vi "Intan_FilterSettings.vi"(0 "VISA resource name":refnum<visa-resource-name>="COM1", 1 "R_L source":u8(ring) items=["ON-chip", "OFF-chip"], 2 "Lower cutoff":u8(ring)=12 items=["10 Hz", "7.5 Hz", "5.0 Hz", "3.0 Hz", "2.5 Hz", "2.0 Hz", "1.5 Hz", "1.0 Hz", "0.75 Hz", "0.5 Hz", "0.3 Hz", "0.25 Hz", "0.10 Hz"], 3 "Upper cutoff":u8(ring)=10 items=["5.0 kHz", "3.0 kHz", "2.5 kHz", "2.0 kHz", "1.5 kHz", "1.0 kHz", "750 Hz", "500 Hz", "300 Hz", "250 Hz", "200 Hz", "150 Hz", "100 Hz"], 4 "error in":errorcluster) -> (5 "VISA resource name out":refnum<visa-resource-name>, 6 "Text response":string, 7 "error out":errorcluster)   [LabVIEW 2015]
doc: "Use this VI to set Intan RHD2000 series BPF filter parameters. If off-chip R_L is selected, then the lower bandwidth depends on the resistor value connected between aux3 and gnd. For GI applications, we typically use 100 Mohm resistor to set 0.01 Hz low cutoff. If on-chip_R_L is selected, then the low cutoff corresponds to the value chosen in the drop-down menu. \n\nBe sure to call the ADC calibrate command after configuring filters.\n\n(Note that there is currently no option to use off-chip RH_1 and RH_2.)"
panel:
  out "ack string":string
  out "string upper":string
  out "string lower":string
  in  "Teensy event char":string="f"
  # "Set BPF cutoffs on RHD2000 chip.\nThis works by sending character 'm' over serial, \nwhich is recognized by Teensy to trigger reading of \ninteger values selected below, then writes the registers 8-13\naccordingly."
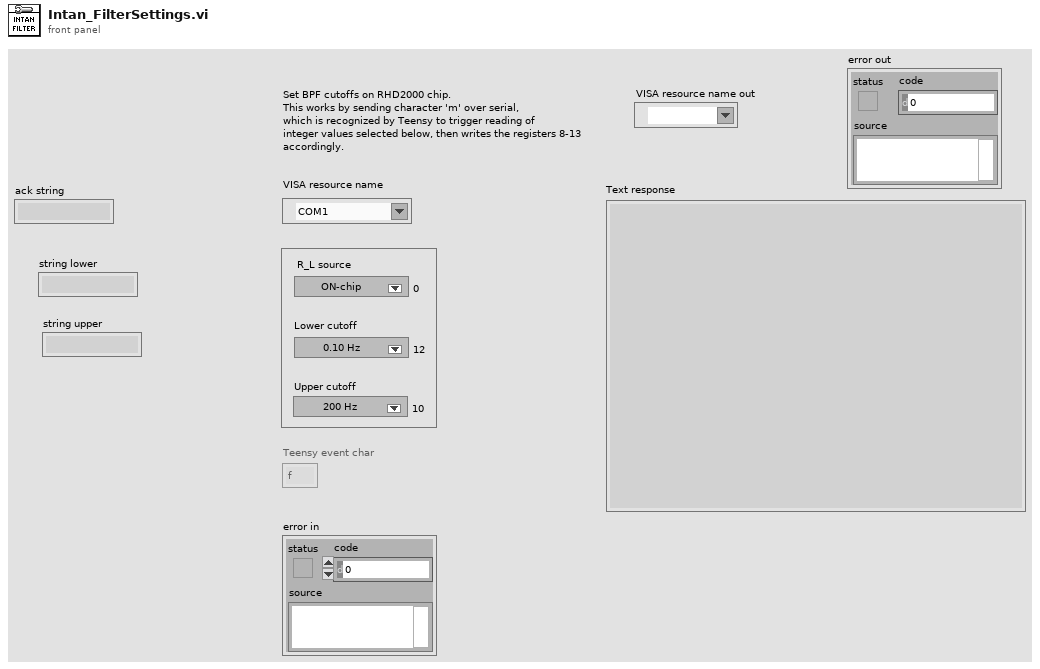
[diagram p1: front panel]
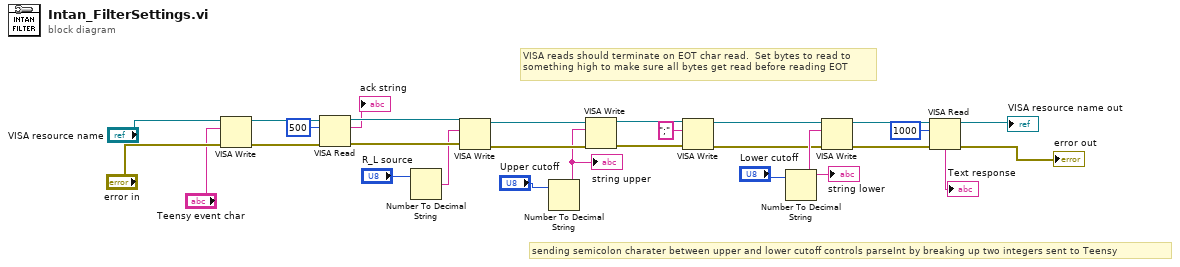
[diagram p0: block diagram]
diagram:
  # "sending semicolon charater between upper and lower cutoff controls parseInt by breaking up two integers sent to Teensy"
  # "VISA reads should terminate on EOT char read.  Set bytes to read to something high to make sure all bytes get read before reading EOT"
  n1 = VISA Write(VISA resource name="VISA resource name", write buffer="Teensy event char", error in (no error)="error in") -> (VISA resource name out=w7:refnum<visa-resource-name>, error out=w6:errorcluster)  [unwired: 1 out]
  n2 = VISA Read(VISA resource name=w7, byte count=u32 500, error in (no error)=w6) -> (VISA resource name out=w25:refnum<visa-resource-name>, read buffer=→"ack string":string, error out=w24:errorcluster)  [unwired: 1 out]
  n3 = Number To Decimal String(number="R_L source") -> (decimal integer string=w15:string)  [unwired: 1 in]
  n4 = VISA Write(VISA resource name=w25, write buffer=w15, error in (no error)=w24) -> (VISA resource name out=w20:refnum<visa-resource-name>, error out=w21:errorcluster)  [unwired: 1 out]
  n5 = Number To Decimal String(number="Upper cutoff") -> (decimal integer string=w14:string)  [unwired: 1 in]
  "string upper" <- w14
  n6 = VISA Write(VISA resource name=w20, write buffer=w14, error in (no error)=w21) -> (VISA resource name out=w13:refnum<visa-resource-name>, error out=w11:errorcluster)  [unwired: 1 out]
  n7 = VISA Write(VISA resource name=w13, write buffer=";", error in (no error)=w11) -> (VISA resource name out=w12:refnum<visa-resource-name>, error out=w10:errorcluster)  [unwired: 1 out]
  n8 = Number To Decimal String(number="Lower cutoff") -> (decimal integer string=w18:string)  [unwired: 1 in]
  "string lower" <- w18
  n9 = VISA Write(VISA resource name=w12, write buffer=w18, error in (no error)=w10) -> (VISA resource name out=w4:refnum<visa-resource-name>, error out=w3:errorcluster)  [unwired: 1 out]
  n10 = VISA Read(VISA resource name=w4, byte count=u32 1000, error in (no error)=w3) -> (VISA resource name out=→"VISA resource name out":refnum<visa-resource-name>, read buffer=→"Text response":string, error out=→"error out":errorcluster)  [unwired: 1 out]
